vi "Search Local Sessions.vi"(8 "error in":errorcluster, 9 "SSH Error":string, 10 "sessions in":string[][](array[string]), 11 "SSH session in":refnum<class "OpenSSH Client.lvclass">) -> (0 "error out":errorcluster, 2 "sessions out":string[][](array[string]), 3 "SSH Error?":bool)   [LabVIEW 2024, in "Session Scanner.lvlib"]
uses:
  Session Scanner.lvlib
  <vilib>/net/SSH/Client/OpenSSH/OpenSSH Client.lvclass
  Support/General Type Defs/Global Data.vi
  Support/General Type Defs/General Type Definitions.lvlib
  <vilib>/net/SSH/NI_SSH.lvlib
  C:/Program Files (x86)/National Instruments/LabVIEW 2024/vi.lib/net/SSH/Client/Generic/Generic Client.lvclass
  C:/Program Files (x86)/National Instruments/LabVIEW 2024/vi.lib/net/SSH/Client/OpenSSH/OpenSSH Client.lvclass
panel:
  out "standard error":string
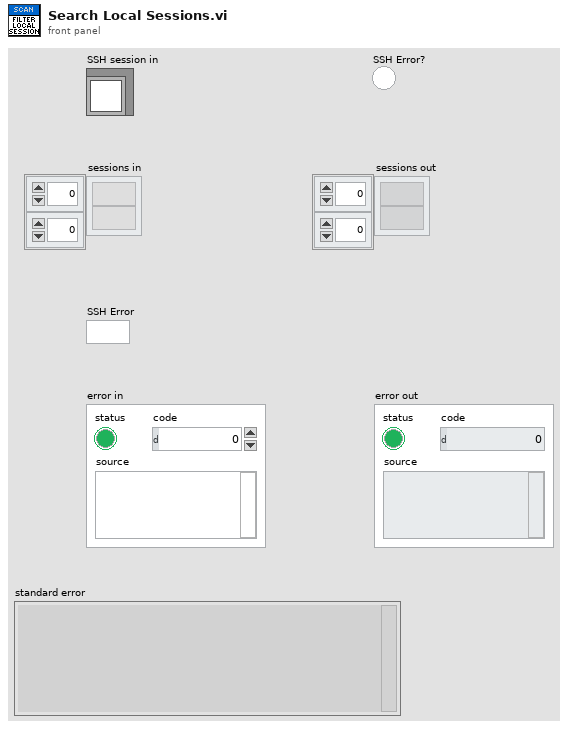
[diagram p1: front panel]
types:
  T1 = typedef "General Type Definitions.lvlib/Device Data.ctl" = cluster{"OS":T2, "User":string, "Password":string, "Hostname":string, "IP Address":string}
  T2 = typedef "General Type Definitions.lvlib/Device OS.ctl" = enum16{"Windows", "Linux"}
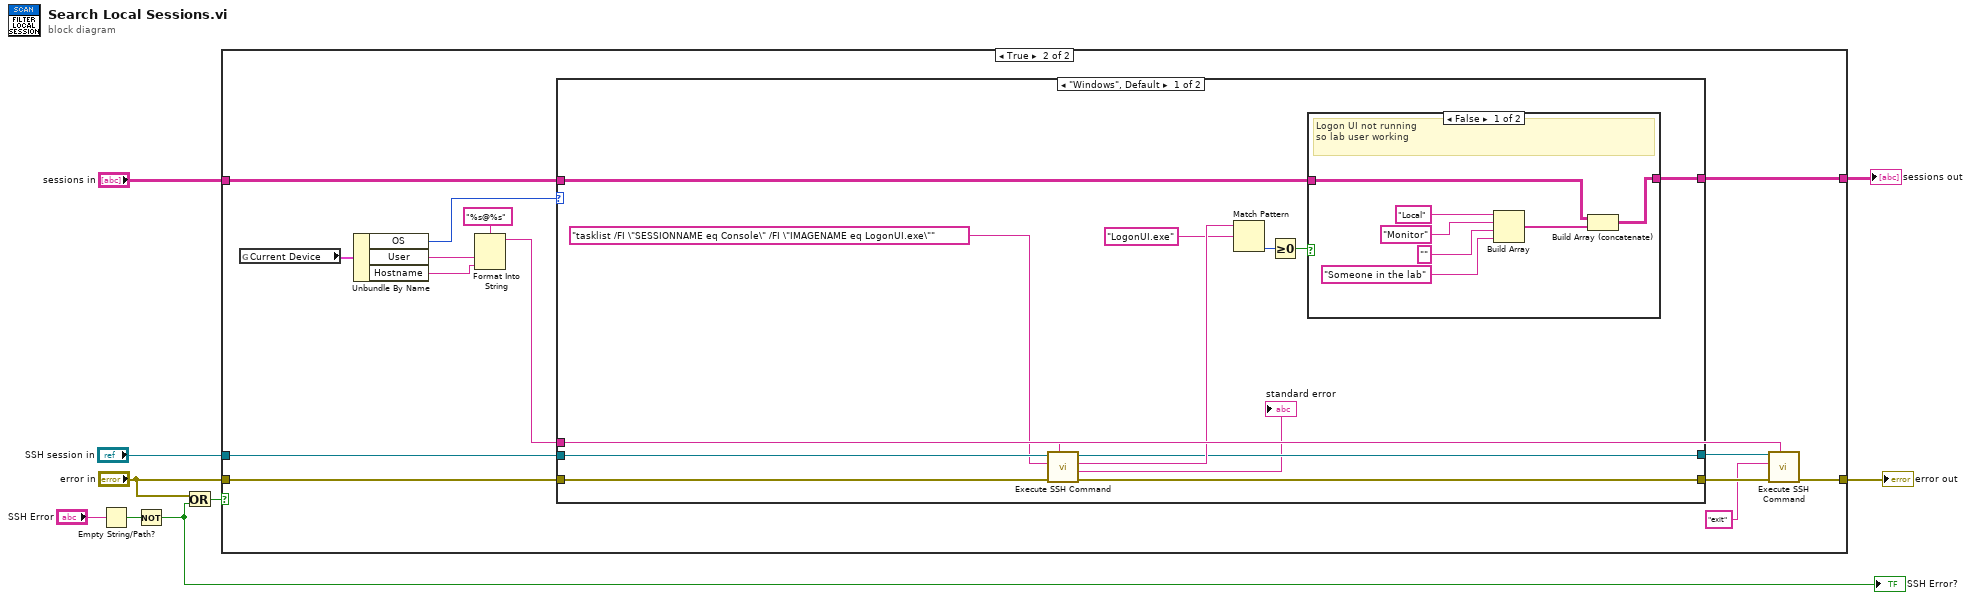
[diagram p0: block diagram]
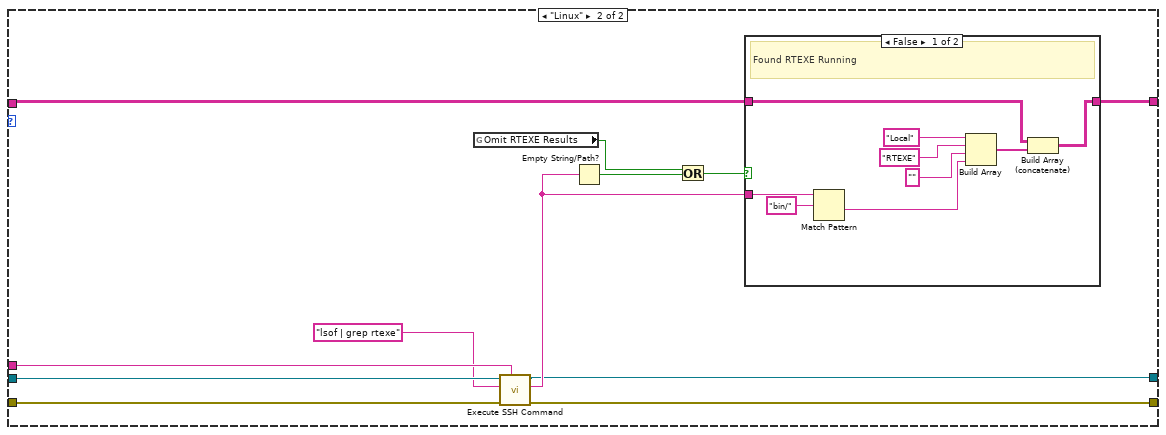
[diagram p4: hidden frame]
diagram:
  n1 = Empty String/Path?(string/path="SSH Error") -> (empty?=w4:bool)
  n2 = Not(x=w4) -> (.not. x?=w1:bool)
  "SSH Error?" <- w1
  n3 = Or(x="error in", y=w1) -> (x .or. y?=w2:bool)
  n4 = case shown="True" w2 {
    tunnel: [w10 w15] -> w9
    tunnel: "sessions in" -> [_ w21]
    tunnel: [_ w20] -> w7
    tunnel: "SSH session in" -> [_ w17]
    tunnel: "error in" -> [w10 w11]
    frame False {
    }
    frame True {
      n5 = global read "Global Data.vi" "Current Device"() -> (w22:T1)
      n6 = Unbundle By Name(w22) -> ("OS"=w18:T2, "User"=w24:string, "Hostname"=w23:string)
      n7 = Format Into String(format string="%s@%s", w24, w23) -> (resulting string=w13:string)  [unwired: 2 in, 1 out]
      n8 = case shown="\"Windows\", Default" w18 {
        tunnel: w21 -> [w37 w50]
        tunnel: [w36 w52] -> w20
        tunnel: w11 -> [w35 w57]
        tunnel: w17 -> [w34 w56]
        tunnel: [w33 w55] -> w16
        tunnel: w13 -> [w32 w54]
        tunnel: [w27 w48] -> w14
        frame "Windows", Default {
          n9 = call <vilib>:"Execute SSH Command.vi"("user@host"=w32, "error in (no error)"=w35, "command line"="tasklist /FI \"SESSIONNAME eq Console\" /FI \"IMAGENAME eq LogonUI.exe\"", "session in"=w34) -> ("error out"=w33:errorcluster, "standard error"=→"standard error":string, "standard output"=w29:string, "session out"=w27:refnum<class "OpenSSH Client.lvclass">)  [unwired: 3 in, 1 out]
          n10 = Match Pattern(string=w29, regular expression="LogonUI.exe") -> (offset past match=w31:i32)  [unwired: 1 in, 3 out]
          n11 = Greater Or Equal To 0?(x=w31) -> (x >= 0?=w30:bool)
          n12 = case shown="False" w30 {
            tunnel: w37 -> [w40 w45]
            tunnel: [w38 w45] -> w36
            frame False {
              # "Logon UI not running\nso lab user working"
              n13 = Build Array("Local", "Monitor" ("element"), "" ("element"), "Someone in the lab" ("element")) -> (w39:string[])
              n14 = Build Array (concatenate)(w40, w39) -> (w38:string[][])
            }
            frame True {
            }
          }
        }
        frame "Linux" {
          n15 = global read "Global Data.vi" "Omit RTEXE Results"() -> (w46:bool)
          n16 = call <vilib>:"Execute SSH Command.vi"("user@host"=w54, "error in (no error)"=w57, "command line"="lsof | grep rtexe", "session in"=w56) -> ("error out"=w55:errorcluster, "standard output"=w49:string, "session out"=w48:refnum<class "OpenSSH Client.lvclass">)  [unwired: 3 in, 2 out]
          n17 = Empty String/Path?(string/path=w49) -> (empty?=w51:bool)
          n18 = Or(x=w46, y=w51) -> (x .or. y?=w47:bool)
          n19 = case shown="False" w47 {
            tunnel: [w62 w67] -> w52
            tunnel: w50 -> [w58 w67]
            tunnel: w49 -> [w61 _]
            frame False {
              # "Found RTEXE Running"
              n20 = Match Pattern(string=w61, regular expression="bin/") -> (after substring=w59:string)  [unwired: 1 in, 3 out]
              n21 = Build Array("Local", "RTEXE" ("element"), "" ("element"), w59) -> (w63:string[])
              n22 = Build Array (concatenate)(w58, w63) -> (w62:string[][])
            }
            frame True {
              # "No RTEXE Running"
            }
          }
        }
      }
      n23 = call <vilib>:"Execute SSH Command.vi"("user@host"=w13, "error in (no error)"=w16, "command line"="exit", "session in"=w14) -> ("error out"=w15:errorcluster)  [unwired: 3 in, 4 out]
    }
  }
  "error out" <- w9
  "sessions out" <- w7
